vi "CUDA Toolkit Read RF Bin quick record 2020 all exec without indicator and warmup.vi"() -> ()   [LabVIEW 2020]
uses:
  Cuda/Source/Methods/Memory Control/CSG/CreateTensor(1DArrayCSG).vi
  Cuda/Source/Methods/Memory Control/SGL/CreateTensor(1DArraySGL).vi
  Cuda/Source/Methods/Memory Control/SGL/HostToDevice(1DArraySGL).vi
  Cuda/Source/Methods/Memory Control/SGL/DeviceToHost&Free(1DArraySGL).vi
  Cuda/Source/Methods/Functions/Numeric/SGL/Divide Array Scalar(SGL).vi
  Cuda/Source/Methods/Functions/CuFFT/FFT C2C(CSG).vi
  Cuda/Source/Methods/Memory Control/CSG/HostToDevice(1DArrayCSG).vi
  Cuda/Source/Methods/Functions/Numeric/SGL/Multiply Array Scalar(SGL).vi
  Cuda/Source/Methods/Functions/Numeric/SGL/Add Array Scalar(SGL).vi
  Cuda/Source/Methods/Memory Control/CSG/DeviceToHost&Free(1DArrayCSG).vi
  Cuda/Source/Methods/Memory Control/SGL/DeviceToHost(1DArraySGL).vi
  Cuda/Source/Tensor.lvclass
panel:
  out "exec time":dbl
  in  "file path":path=path "E:/TEMP.BIN"
  out "Intensity Chart":sgl[][](graph)
  out "Waveform Graph":sgl[](graph)
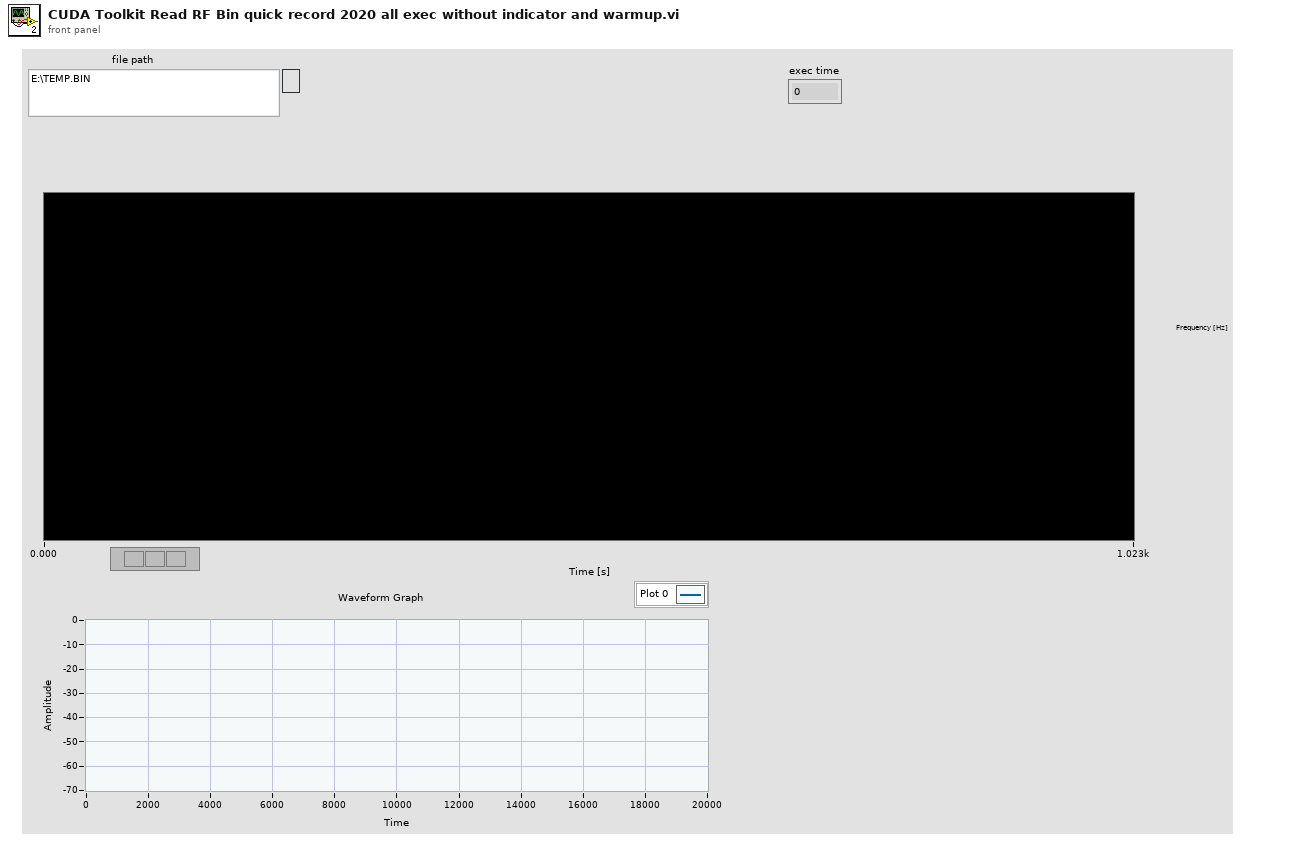
[diagram p1: front panel]
types:
  T1 = enum16{"open", "replace", "create", "open or create", "replace or create", "replace or create with confirmation"}
  T2 = enum16{"big-endian, network order", "native, host order", "little-endian"}
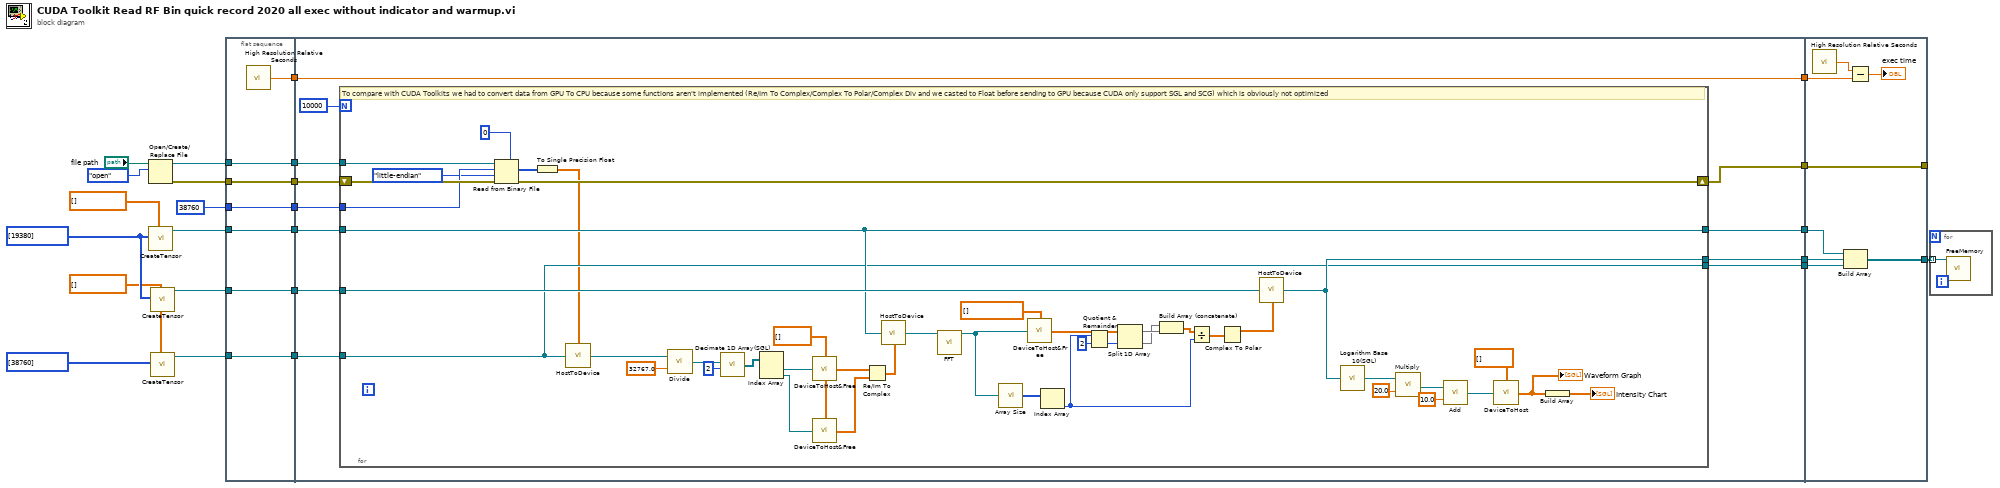
[diagram p0: block diagram]
diagram:
  w6 = sgl[] [] ("element")
  w7 = i32[] [19380] ("count (1)")
  n1 = Open/Create/Replace File(file path (use dialog)="file path", operation (0:open)=T1."open") -> (refnum out=w23:refnum<file>, error out=w11:errorcluster)  [unwired: 4 in, 1 out]
  n2 = call-poly "CreateTensor.vi"("type"=csg[] [] ("element"), "shape"=w7) -> ("Tensor out"=w10:refnum<class "Tensor.lvclass">)  [unwired: 8 in, 1 out]
  n3 = call-poly "CreateTensor.vi"("type"=w6, "shape"=w7) -> ("Tensor out"=w21:refnum<class "Tensor.lvclass">)  [unwired: 8 in, 1 out]
  n4 = call-poly "CreateTensor.vi"("type"=w6, "shape"=i32[] [38760] ("count (1)")) -> ("Tensor out"=w22:refnum<class "Tensor.lvclass">)  [unwired: 8 in, 1 out]
  n5 = flat-sequence {
    tunnel: 38760 ("count (1)") -> [w28]
    tunnel: w21 -> [w29]
    tunnel: w10 -> [w30]
    tunnel: w22 -> [w31]
    tunnel: w23 -> [w32]
    tunnel: [w32] -> w20
    tunnel: [w31] -> w19
    tunnel: [w30] -> w18
    tunnel: [w29] -> w17
    tunnel: [w28] -> w16
    tunnel: [w27] -> w14
    tunnel: [w26] -> w12
    tunnel: w11 -> [w26]
    tunnel: w20 -> [w43]
    tunnel: w19 -> [w42]
    tunnel: w18 -> [w41]
    tunnel: w17 -> [w40]
    tunnel: w16 -> [w39]
    tunnel: [w38] -> w15
    tunnel: w14 -> [w37]
    tunnel: [w37] -> w13
    tunnel: w12 -> [w36]
    tunnel: [w35] -> w4
    tunnel: [w34] -> w3
    tunnel: [w33] -> w2
    tunnel: [w96] -> _
    tunnel: w15 -> [w96]
    tunnel: w13 -> [w94]
    tunnel: w4 -> [w92]
    tunnel: w3 -> [w91]
    tunnel: w2 -> [w90]
    tunnel: [w89] -> w1
    frame #0 {
      n6 = call <vilib>:"High Resolution Relative Seconds.vi"() -> ("relative seconds"=w27:dbl)
    }
    frame #1 {
      n7 = for {
        N: 10000 -> [_]
        shift-right: [w84] -> w38
        shift-left: w36 -> [w88]
        tunnel: w43 -> [w87]
        tunnel: w42 -> [w54]
        tunnel: w39 -> [w86]
        tunnel: w41 -> [w56]
        tunnel: w40 -> [w85]
        tunnel: [w56] -> w35
        tunnel: [w55] -> w34
        tunnel: [w54] -> w33
        w57 = sgl[] [] ("type")
        # "To compare with CUDA Toolkits we had to convert data from GPU To CPU because some functions aren't implemented (Re/Im To Complex/Complex To Polar/Complex Div and we casted to Float before sending to GPU because CUDA only support SGL and SCG) which is obviously not optimized"
        n8 = Read from Binary File(5:i16 0 ("Numeric"), 8:w88, 9:T2."little-endian" ("byte order (0:big-endian, network order)"), 10:w86, 11:w87) -> (0:w84:errorcluster, 2:w80:i16[])  [unwired: 1 in, 2 out]
        n9 = To Single Precision Float(number=w80) -> (single precision float=w46:sgl[])
        n10 = call-poly "HostToDevice.vi"("data"=w46, "Tensor in"=w54) -> ("Tensor out"=w79:refnum<class "Tensor.lvclass">)  [unwired: 13 in]
        n11 = call-poly "Divide.vi"("y"=sgl 32767.0 ("Numeric"), "x"=w79) -> ("x / y"=w62:refnum<class "Tensor.lvclass">)
        n12 = call "Decimate 1D Array(SGL).vi"("nb_output_array"=2, "array"=w62) -> ("decimated arrays"=w65:refnum<class "Tensor.lvclass">[])  [unwired: 4 in]
        n13 = Index Array(array=w65) -> (element #1=w63:refnum<class "Tensor.lvclass">, element #2=w64:refnum<class "Tensor.lvclass">)  [unwired: 2 in]
        n14 = call-poly "DeviceToHost&Free.vi"("type"=w57, "Tensor in"=w63) -> ("data"=w71:sgl[])  [unwired: 13 in]
        n15 = call-poly "DeviceToHost&Free.vi"("type"=w57, "Tensor in"=w64) -> ("data"=w70:sgl[])  [unwired: 13 in]
        n16 = Re/Im To Complex(1:w70, 2:w71) -> (0:w60:csg[])
        n17 = call-poly "HostToDevice.vi"("data"=w60, "Tensor in"=w56) -> ("Tensor out"=w69:refnum<class "Tensor.lvclass">)  [unwired: 13 in]
        n18 = call-poly "FFT.vi"("x"=w69) -> ("y"=w59:refnum<class "Tensor.lvclass">)  [unwired: 9 in, 1 out]
        n19 = call "Array Size.vi"("array"=w59) -> ("size(s)"=w78:i32[])
        n20 = call-poly "DeviceToHost&Free.vi"("type"=csg[] [], "Tensor in"=w59) -> ("data"=w53:csg[])  [unwired: 13 in]
        n21 = Index Array(array=w78) -> (element=w52:i32)  [unwired: 1 in]
        n22 = Quotient & Remainder(x=w52, y=2) -> (floor(x/y)=w51:i32)  [unwired: 1 out]
        n23 = Split 1D Array(array=w53, index=w51) -> (first subarray=w49:csg[], second subarray=w48:csg[])
        n24 = Build Array (concatenate)(w48, w49) -> (w47:csg[])
        n25 = Divide(x=w47, y=w52) -> (x/y=w58:csg[])
        n26 = Complex To Polar(r * e^(i*theta)=w58) -> (r=w61:sgl[])  [unwired: 1 out]
        n27 = call-poly "HostToDevice.vi"("data"=w61, "Tensor in"=w85) -> ("Tensor out"=w55:refnum<class "Tensor.lvclass">)  [unwired: 13 in]
        n28 = call "Logarithm Base 10(SGL).vi"("x"=w55) -> ("log(x)"=w77:refnum<class "Tensor.lvclass">)
        n29 = call-poly "Multiply.vi"("y"=sgl 20.0 ("Numeric"), "x"=w77) -> ("x * y"=w74:refnum<class "Tensor.lvclass">)
        n30 = call-poly "Add.vi"("y"=sgl 10.0 ("Numeric"), "x"=w74) -> ("x + y"=w67:refnum<class "Tensor.lvclass">)
        n31 = call-poly "DeviceToHost.vi"("type"=sgl[] [], "Tensor in"=w67) -> ("data"=w45:sgl[])  [unwired: 13 in]
        "Waveform Graph" <- w45
        n32 = Build Array(w45) -> (→"Intensity Chart":sgl[][])
      }
    }
    frame #2 {
      n33 = call <vilib>:"High Resolution Relative Seconds.vi"() -> ("relative seconds"=w95:dbl)
      n34 = Build Array(w92, w91, w90) -> (w89:refnum<class "Tensor.lvclass">[])
      n35 = Subtract(x=w95, y=w94) -> (x-y=→"exec time":dbl)
    }
  }
  n36 = for {
    tunnel: w1 -> [w97] mode=indexing
    n37 = call "FreeMemory.vi"("Tensor in"=w97) -> ()  [unwired: 10 in, 1 out]
  }
